vi "icListenHF.vi"() -> ()   [LabVIEW 2020]
uses:
  SubVIs/PAM Reset Array.vi
  SubVIs/icListen 3 Reset.vi
  SubVIs/icListen 2 Reset.vi
  SubVIs/icListen 4 Reset.vi
  SubVIs/icListen 1 Reset.vi
  SubVIs/icListen 2 Connected.vi
  SubVIs/icListen 4 Connected.vi
  SubVIs/icListen 3 Connected.vi
  SubVIs/icListen 1 Connected.vi
  SubVIs/icListen 3 Enabled.vi
  SubVIs/icListen 2 Enabled.vi
  SubVIs/icListen 4 Enabled.vi
  SubVIs/icListen 1 Enabled.vi
  SubVIs/icListen 2 Initialized.vi
  SubVIs/icListen 4 Initialized.vi
  SubVIs/icListen 3 Initialized.vi
  SubVIs/icListen 1 Initialized.vi
  SubVIs/icListen 4 Synchronization.vi
  SubVIs/icListen 3 Synchronization.vi
  SubVIs/icListen 2 Synchronization.vi
  SubVIs/icListen 1 Synchronization.vi
  SubVIs/icListen 4 Serial Number.vi
  SubVIs/icListen 3 Serial Number.vi
  SubVIs/icListen 2 Serial Number.vi
  SubVIs/icListen 1 Serial Number.vi
  SubVIs/PAM Sample Rate.vi
  SubVIs/icListen 1 Position.vi
  SubVIs/icListen 2 Position.vi
  SubVIs/icListen 3 Position.vi
  SubVIs/icListen 4 Position.vi
  SubVIs/PAM Array Buffer Size.vi
  SubVIs/icListen 1 Response.vi
  SubVIs/icListen 2 Response.vi
  SubVIs/icListen 3 Response.vi
  SubVIs/icListen 1 Metadata.vi
  SubVIs/icListen 2 Metadata.vi
  SubVIs/icListen 3 Metadata.vi
  SubVIs/icListen 4 Response.vi
  SubVIs/icListen 4 Metadata.vi
  PAM Library.lvlib
  SubVIs/PAM Volts per Bit.vi
panel:
  out "SN 4":string
  out "SN 3":string
  out "SN 2":string
  out "SN 1":string
  in  "Pos 4":string="Aft Right"
  in  "Pos 3":string="Aft Left"
  in  "Pos 2":string="Fore Right"
  in  "Pos 1":string="Fore Left"
  in  "Sample Rate":T1(ring)=enum."512000"
  in  "Stop":bool
  out "Y min":dbl format="%0.2f"
  out "Y max":dbl format="%0.2f"
  out "size(s) 2":i32
  out "size(s)":i32
  out "Waveform Chart":waveform(dbl)(graph)
  out "Error Out 2":errorcluster
  in  "Error In":errorcluster
  out "TCP IDs 4":T2
  in  "Reset\nArray":bool
  in  "Enable icListen 4":bool
  in  "Enable icListen 3":bool
  in  "Enable icListen 2":bool
  in  "Enable icListen 1":bool=TRUE
  out "Temp":dbl format="%.1g"
  out "Time":string
  out "Status":string="Disabled"
  out "Date":string
  out "Humid":dbl format="%.1g"
  in  "Reset \nicListen 4":bool
  out "Temp":dbl format="%.1g"
  out "Time":string
  out "Temp":dbl format="%.1g"
  out "Time":string
  out "Status":string="Disabled"
  out "Status":string="Disabled"
  out "Temp":dbl format="%.1g"
  out "Time":string
  out "Date":string
  out "Date":string
  out "Date":string
  out "Humid":dbl format="%.1g"
  out "Humid":dbl format="%.1g"
  out "Humid":dbl format="%.1g"
  out "Status":string="Disabled"
  in  "Reset \nicListen 3":bool
  in  "Reset \nicListen 2":bool
  out "TCP IDs 3":T2
  out "TCP IDs 2":T2
  out "Display":waveform(dbl)[](graph)
  out "TCP IDs 1":T2
  out "Error Out":errorcluster
  out "Reset Varibles":errorcluster
  in  "Reset \nicListen 1":bool
  # "Hydrophone Array"
  # "Status & Controls"
  # "Sample Rate [Hz]"
  # "Position"
  # "Status"
  # "Time"
  # "Date"
  # "Temp."
  # "Humid."
  # "SN"
  # "icListen 1"
  # "icListen 2"
  # "icListen 3"
  # "icListen 4"
  # "icListen 1 (SN 1243, Fore Left)"
  # "icListen 2 (SN 1243, Fore Right)"
  # "icListen 3 (SN 1242, Aft Left)"
  # "icListen 4 (SN 1244, Aft Right)"
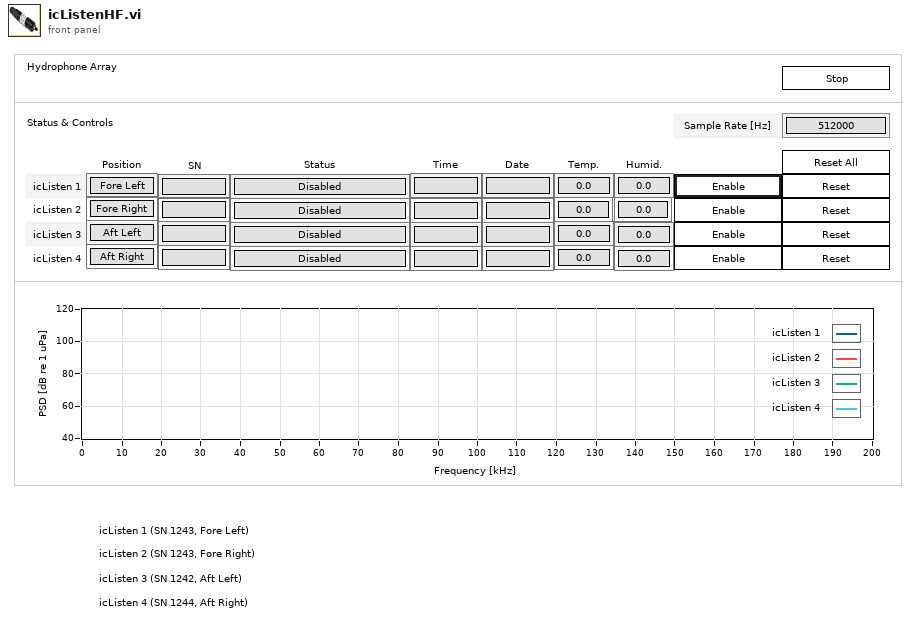
[diagram p1: front panel]
types:
  T1 = enum32{"16000", "32000", "64000", "128000", "256000", "512000"}
  T2 = cluster{"CC Id":refnum<k5>, "Waveform ID":refnum<k5>, "Spectrum ID":refnum<k5>, "Other Data ID":refnum<k5>}
  T3 = cluster{"default (0 U32) 2":i16, "default (0 U32)":i32, "unsigned 64bit integer":u64}
  T4 = cluster{"System Time Status":u8, "Sync Status":u8, "PPS Count":u32, "Sync Offset":u32}
  T5 = cluster{"default (0 U32) 2":i16, "default (0 U32)":i32, "unsigned 64bit integer":u64}[]
  T6 = cluster{"Date":string, "Time":string, "Temperature":dbl, "Humidity":dbl, "Battery Charge":i32}
  T7 = cluster{"State":enum16{"Align with Stream", "Read Header Byte", "Read Data Header", "Read Event Header", "Read Notification", "Read Data"}, "Sample Count":i32, "Timestamp":u64, "Payload":u16, "Repeated Error":i32, "Header Byte":string}
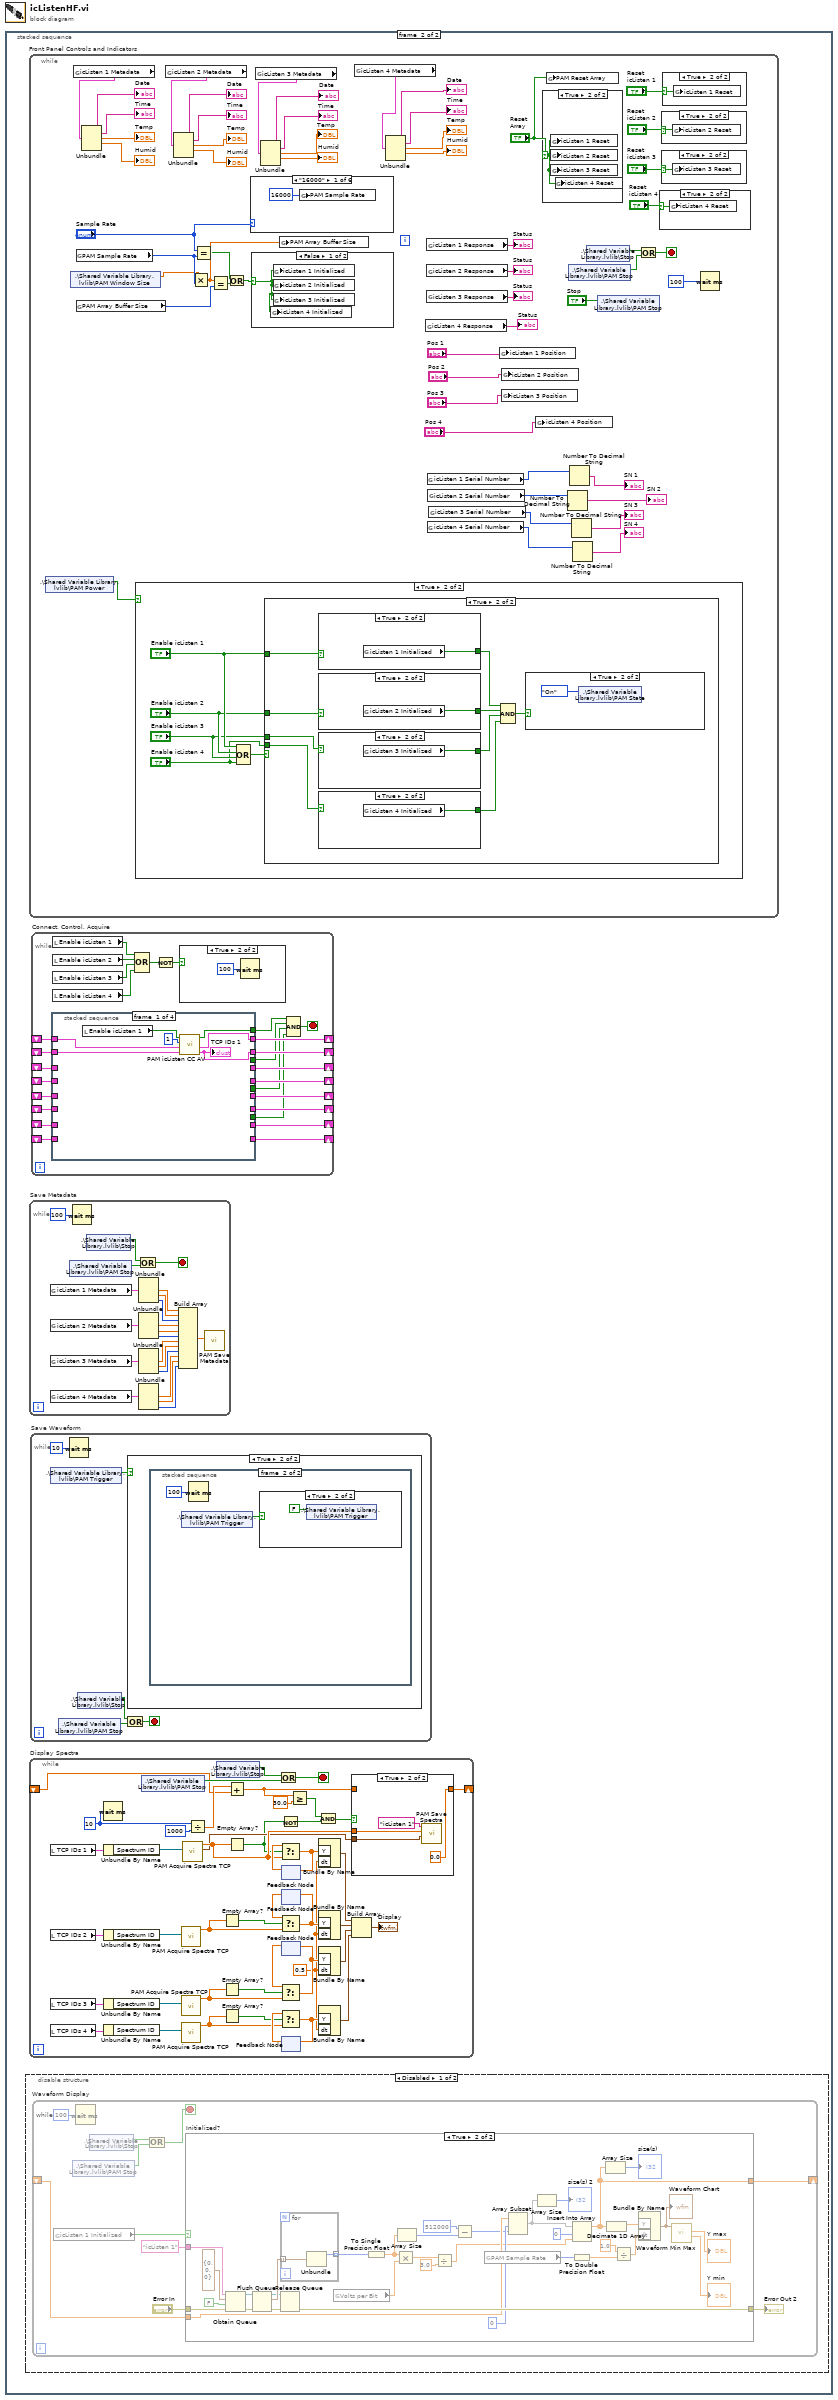
[diagram p0: block diagram]
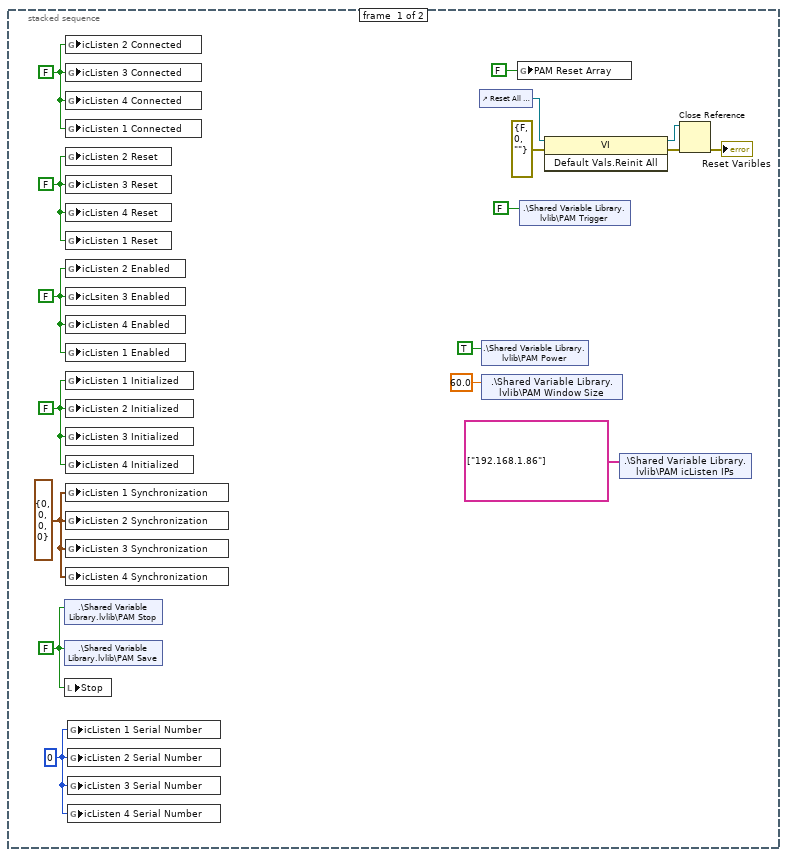
[diagram p2: hidden frame]
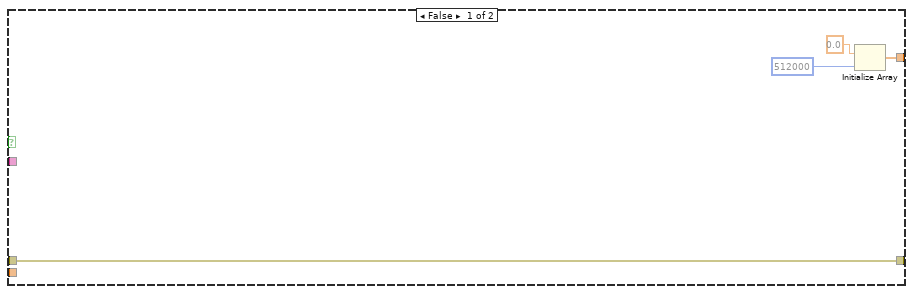
[diagram p4: hidden frame]
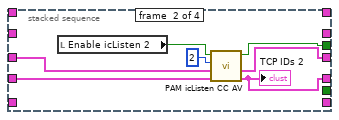
[diagram p7: hidden frame]
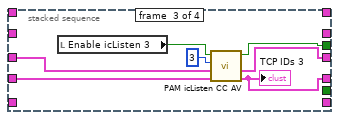
[diagram p8: hidden frame]
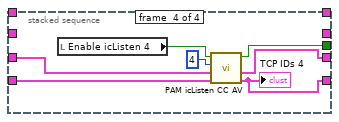
[diagram p9: hidden frame]
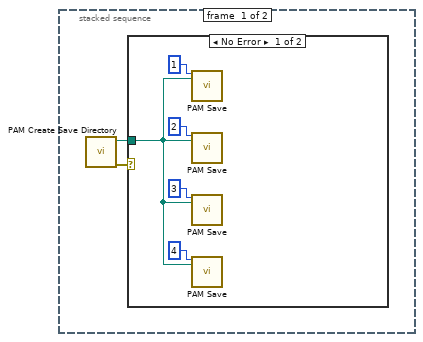
[diagram p11: hidden frame]
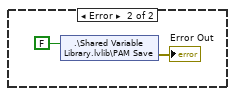
[diagram p12: hidden frame]
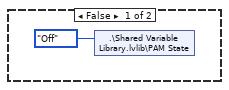
[diagram p14: hidden frame]
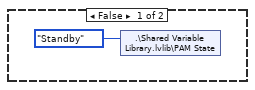
[diagram p15: hidden frame]
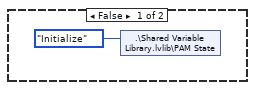
[diagram p16: hidden frame]
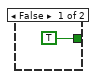
[diagram p17: hidden frame]
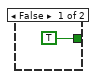
[diagram p18: hidden frame]
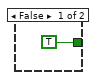
[diagram p19: hidden frame]
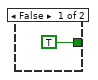
[diagram p20: hidden frame]
diagram:
  n1 = stacked-sequence {
    frame #0 {
      w4 = u16 0 ("icListen 1 Serial Number")
      w6 = FALSE ("PAM Save")
      w8 = T4 {"System Time Status"=0, "Sync Status"=0, "PPS Count"=0, "Sync Offset"=0} ("icListen 1 Synchronization")
      w13 = FALSE ("PAM Stop VI")
      w12 = FALSE ("PAM Stop VI")
      w11 = FALSE ("PAM Stop VI")
      w10 = FALSE ("PAM Stop VI")
      n2 = shared-variable ".\\Shared Variable Library.lvlib\\PAM Stop"(w6) -> ()  [unwired: 1 in, 1 out]
      n3 = shared-variable ".\\Shared Variable Library.lvlib\\PAM Save"(w6) -> ()  [unwired: 1 in, 1 out]
      n4 = local write "Stop"(w6) -> ()
      n5 = global write "icListen 2 Connected.vi" "icListen 2 Connected"(w11) -> ()
      n6 = global write "icListen 3 Connected.vi" "icListen 3 Connected"(w11) -> ()
      n7 = global write "icListen 4 Connected.vi" "icListen 4 Connected"(w11) -> ()
      n8 = global write "icListen 1 Connected.vi" "icListen 1 Connected"(w11) -> ()
      n9 = global write "icListen 2 Reset.vi" "icListen 2 Reset"(w10) -> ()
      n10 = global write "icListen 3 Reset.vi" "icListen 3 Reset"(w10) -> ()
      n11 = global write "icListen 4 Reset.vi" "icListen 4 Reset"(w10) -> ()
      n12 = global write "icListen 1 Reset.vi" "icListen 1 Reset"(w10) -> ()
      n13 = global write "icListen 2 Enabled.vi" "icListen 2 Enabled"(w12) -> ()
      n14 = global write "icListen 3 Enabled.vi" "icLsiten 3 Enabled"(w12) -> ()
      n15 = global write "icListen 4 Enabled.vi" "icListen 4 Enabled"(w12) -> ()
      n16 = global write "icListen 1 Enabled.vi" "icListen 1 Enabled"(w12) -> ()
      n17 = global write "icListen 1 Initialized.vi" "icListen 1 Initialized"(w13) -> ()
      n18 = global write "icListen 2 Initialized.vi" "icListen 2 Initialized"(w13) -> ()
      n19 = global write "icListen 3 Initialized.vi" "icListen 3 Initialized"(w13) -> ()
      n20 = global write "icListen 4 Initialized.vi" "icListen 4 Initialized"(w13) -> ()
      n21 = global write "icListen 1 Synchronization.vi" "icListen 1 Synchronization"(w8) -> ()
      n22 = global write "icListen 2 Synchronization.vi" "icListen 2 Synchronization"(w8) -> ()
      n23 = global write "icListen 3 Synchronization.vi" "icListen 3 Synchronization"(w8) -> ()
      n24 = global write "icListen 4 Synchronization.vi" "icListen 4 Synchronization"(w8) -> ()
      n25 = global write "icListen 1 Serial Number.vi" "icListen 1 Serial Number"(w4) -> ()
      n26 = global write "icListen 2 Serial Number.vi" "icListen 2 Serial Number"(w4) -> ()
      n27 = global write "icListen 3 Serial Number.vi" "icListen 3 Serial Number"(w4) -> ()
      n28 = global write "icListen 4 Serial Number.vi" "icListen 4 Serial Number"(w4) -> ()
      n29 = control-ref of="Reset All VI Variables"() -> (w14:refnum<vi>)
      n30 = shared-variable ".\\Shared Variable Library.lvlib\\PAM Power"(TRUE ("PAM Power")) -> ()  [unwired: 1 in, 1 out]
      n31 = shared-variable ".\\Shared Variable Library.lvlib\\PAM Window Size"(60.0 ("PAM Window Size")) -> ()  [unwired: 1 in, 1 out]
      n32 = global write "PAM Reset Array.vi" "PAM Reset Array"(FALSE ("PAM Stop VI")) -> ()
      n33 = shared-variable ".\\Shared Variable Library.lvlib\\PAM Trigger"(FALSE ("PAM Trigger")) -> ()  [unwired: 1 in, 1 out]
      n34 = invoke class="VI" method="Default Vals.Reinit All"(reference=w14, error in=errorcluster {"status"=FALSE, "code"=0, "source"=""} ("error in (no error)")) -> (reference out=w9:refnum<vi>, error out=w17:errorcluster)  [unwired: 1 in, 1 out]
      n35 = shared-variable ".\\Shared Variable Library.lvlib\\PAM icListen IPs"(string[] ["192.168.1.86"] ("PAM icListen IPs")) -> ()  [unwired: 1 in, 1 out]
      n36 = Close Reference(reference=w9, error in (no error)=w17) -> (error out=→"Reset Varibles":errorcluster)
    }
    frame #1 {
      n37 = disable-structure shown="Disabled" {
        frame Disabled {
          n38 = while "Waveform Display" {
            shift-right: [w73] -> _
            shift-left: _ -> [w72]
            stop <- w74 stop-if-true
            n39 = global read "icListen 1 Initialized.vi" "icListen 1 Initialized"() -> (w69:bool)
            n40 = shared-variable ".\\Shared Variable Library.lvlib\\PAM Stop"() -> (w75:bool)  [unwired: 1 in, 1 out]
            n41 = Wait (ms)(milliseconds to wait=u32 100) -> ()  [unwired: 1 out]
            n42 = shared-variable ".\\Shared Variable Library.lvlib\\Stop"() -> (w76:bool)  [unwired: 1 in, 1 out]
            n43 = Compound Arithmetic op=OR(w76, w75) -> (w74:bool)
            n44 = case "Initialized?" shown="True" w69 {
              tunnel: "Error In" -> [w80 w109]
              tunnel: [w80 w98] -> w71
              tunnel: "icListen 1" ("name (unnamed)") -> [_ w114]
              tunnel: [w77 w85] -> w73
              tunnel: w72 -> [_ w97]
              frame False {
                n45 = Initialize Array(0.0, 512000 ("index")) -> (w77:dbl[])
              }
              frame True {
                n46 = Obtain Queue(name (unnamed)=w114, element data type=T3 {"default (0 U32) 2"=0, "default (0 U32)"=0, "unsigned 64bit integer"=0} ("output cluster"), create if not found? (T)=FALSE, error in (no error)=w109) -> (queue out=w107:refnum<queue>, error out=w106:errorcluster)  [unwired: 1 in, 1 out]
                n47 = Flush Queue(queue=w107, error in (no error)=w106) -> (queue out=w100:refnum<queue>, remaining elements=w102:T5, error out=w99:errorcluster)
                n48 = for {
                  tunnel: w102 -> [w116] mode=indexing
                  tunnel: [w115] -> w103 mode=indexing
                  n49 = Unbundle(w116) -> ("default (0 U32) 2"=w115:i16)  [unwired: 2 out]
                }
                n50 = Release Queue(queue=w100, error in (no error)=w99) -> (error out=w98:errorcluster)  [unwired: 1 in, 2 out]
                n51 = global read "PAM Volts per Bit.vi" "Volts per Bit"() -> (w104:dbl)
                n52 = To Single Precision Float(number=w103) -> (single precision float=w95:sgl[])
                n53 = Multiply(x=w95, y=w104) -> (x*y=w96:dbl[])
                n54 = Array Size(array=w95) -> (size(s)=w92:i32)
                n55 = Divide(x=w96, y=3.0) -> (x/y=w87:dbl[])
                n56 = Subtract(x=512000 ("index"), y=w92) -> (x-y=w91:i32)
                n57 = global read "PAM Sample Rate.vi" "PAM Sample Rate"() -> (w108:i32)
                n58 = Array Subset(array=w97, index=0, length=w91) -> (w89:dbl[])
                n59 = Array Size(array=w89) -> (size(s)=→"size(s) 2":i32)
                n60 = Insert Into Array(array=w89, index=0, new element=w87) -> (w85:dbl[])
                n61 = To Double Precision Float(number=w108) -> (double precision float=w112:dbl)
                n62 = Array Size(array=w85) -> (size(s)=→"size(s)":i32)
                n63 = Decimate 1D Array(w85) -> (w84:dbl[])  [unwired: 1 out]
                n64 = Divide(x=1.0, y=w112) -> (x/y=w113:dbl)
                n65 = Bundle By Name("Y"=w84, "dt"=w113) -> (w83:waveform(dbl))  [unwired: 1 in]
                "Waveform Chart" <- w83
                n66 = call <vilib>:"Waveform Min Max.vi"("waveform in"=w83) -> ("Y min"=→"Y min":dbl, "Y max"=→"Y max":dbl)  [unwired: 5 in, 4 out]
              }
            }
            "Error Out 2" <- w71
          }
        }
        frame Enabled {
        }
      }
      n67 = while "Front Panel Controls and Indicators" {
        stop <- w234 stop-if-true
        n68 = shared-variable ".\\Shared Variable Library.lvlib\\PAM Power"() -> (w224:bool)  [unwired: 1 in, 1 out]
        n69 = shared-variable ".\\Shared Variable Library.lvlib\\PAM Window Size"() -> (w223:dbl)  [unwired: 1 in, 1 out]
        n70 = global read "icListen 1 Metadata.vi" "icListen 1 Metadata"() -> (w242:T6)
        n71 = global read "PAM Sample Rate.vi" "PAM Sample Rate"() -> (w251:i32)
        n72 = global read "PAM Array Buffer Size.vi" "PAM Array Buffer Size"() -> (w263:i32)
        n73 = Unbundle(w242) -> ("Date"=→"Date":string, "Time"=→"Time":string, "Temperature"=→"Temp":dbl, "Humidity"=→"Humid":dbl)  [unwired: 1 out]
        n74 = case shown="True" w224 {
          frame False {
            n75 = shared-variable ".\\Shared Variable Library.lvlib\\PAM State"(enum16{"Off", "Initialize", "On", "Standby"}."Off" ("PAM State")) -> ()  [unwired: 1 in, 1 out]
          }
          frame True {
            n76 = Compound Arithmetic op=OR("Enable icListen 1", "Enable icListen 2", "Enable icListen 3", "Enable icListen 4") -> (w267:bool)
            n77 = case shown="True" w267 {
              tunnel: "Enable icListen 1" -> [_ w281]
              tunnel: "Enable icListen 2" -> [_ w280]
              tunnel: "Enable icListen 3" -> [_ w279]
              tunnel: "Enable icListen 4" -> [_ w278]
              frame False {
                n78 = shared-variable ".\\Shared Variable Library.lvlib\\PAM State"(enum16{"Off", "Initialize", "On", "Standby"}."Standby" ("PAM State")) -> ()  [unwired: 1 in, 1 out]
              }
              frame True {
                n79 = case shown="True" w281 {
                  tunnel: [TRUE ("icListen 1 Initialized") w291] -> w276
                  frame False {
                  }
                  frame True {
                    n80 = global read "icListen 1 Initialized.vi" "icListen 1 Initialized"() -> (w291:bool)
                  }
                }
                n81 = case shown="True" w280 {
                  tunnel: [TRUE ("icListen 1 Initialized") w289] -> w275
                  frame False {
                  }
                  frame True {
                    n82 = global read "icListen 2 Initialized.vi" "icListen 2 Initialized"() -> (w289:bool)
                  }
                }
                n83 = case shown="True" w279 {
                  tunnel: [TRUE ("icListen 1 Initialized") w287] -> w274
                  frame False {
                  }
                  frame True {
                    n84 = global read "icListen 3 Initialized.vi" "icListen 3 Initialized"() -> (w287:bool)
                  }
                }
                n85 = case shown="True" w278 {
                  tunnel: [TRUE ("icListen 1 Initialized") w285] -> w273
                  frame False {
                  }
                  frame True {
                    n86 = global read "icListen 4 Initialized.vi" "icListen 4 Initialized"() -> (w285:bool)
                  }
                }
                n87 = Compound Arithmetic op=AND(w276, w275, w274, w273) -> (w277:bool)
                n88 = case shown="True" w277 {
                  frame False {
                    n89 = shared-variable ".\\Shared Variable Library.lvlib\\PAM State"(enum16{"Off", "Initialize", "On", "Standby"}."Initialize" ("PAM State")) -> ()  [unwired: 1 in, 1 out]
                  }
                  frame True {
                    n90 = shared-variable ".\\Shared Variable Library.lvlib\\PAM State"(enum16{"Off", "Initialize", "On", "Standby"}."On" ("PAM State")) -> ()  [unwired: 1 in, 1 out]
                  }
                }
              }
            }
          }
        }
        n91 = global read "icListen 2 Metadata.vi" "icListen 2 Metadata"() -> (w243:T6)
        n92 = Unbundle(w243) -> ("Date"=→"Date":string, "Time"=→"Time":string, "Temperature"=→"Temp":dbl, "Humidity"=→"Humid":dbl)  [unwired: 1 out]
        n93 = Multiply(x=w223, y=w251) -> (x*y=w264:dbl)
        n94 = Equal?(x="Sample Rate", y=w251) -> (x = y?=w262:bool)
        n95 = Equal?(x=w264, y=w263) -> (x = y?=w260:bool)
        n96 = Or(x=w262, y=w260) -> (x .or. y?=w261:bool)
        n97 = case shown="\"16000\"" "Sample Rate" {
          frame "16000" {
            n98 = global write "PAM Sample Rate.vi" "PAM Sample Rate"(16000 ("PAM Sample Rate")) -> ()
          }
          frame "32000" {
            n99 = global write "PAM Sample Rate.vi" "PAM Sample Rate"(32000 ("PAM Sample Rate")) -> ()
          }
          frame "64000", Default {
            n100 = global write "PAM Sample Rate.vi" "PAM Sample Rate"(64000 ("PAM Sample Rate")) -> ()
          }
          frame "128000" {
            n101 = global write "PAM Sample Rate.vi" "PAM Sample Rate"(128000 ("PAM Sample Rate")) -> ()
          }
          frame "256000" {
            n102 = global write "PAM Sample Rate.vi" "PAM Sample Rate"(256000 ("PAM Sample Rate")) -> ()
          }
          frame "512000" {
            n103 = global write "PAM Sample Rate.vi" "PAM Sample Rate"(512000 ("PAM Sample Rate")) -> ()
          }
        }
        n104 = case shown="False" w261 {
          selector: w261 -> [w297 _]
          frame False {
            n105 = global write "icListen 4 Initialized.vi" "icListen 4 Initialized"(w297) -> ()
            n106 = global write "icListen 1 Initialized.vi" "icListen 1 Initialized"(w297) -> ()
            n107 = global write "icListen 2 Initialized.vi" "icListen 2 Initialized"(w297) -> ()
            n108 = global write "icListen 3 Initialized.vi" "icListen 3 Initialized"(w297) -> ()
          }
          frame True {
          }
        }
        n109 = global read "icListen 3 Metadata.vi" "icListen 3 Metadata"() -> (w244:T6)
        n110 = Unbundle(w244) -> ("Date"=→"Date":string, "Time"=→"Time":string, "Temperature"=→"Temp":dbl, "Humidity"=→"Humid":dbl)  [unwired: 1 out]
        n111 = global write "PAM Array Buffer Size.vi" "PAM Array Buffer Size"(w264) -> ()
        n112 = global read "icListen 4 Metadata.vi" "icListen 4 Metadata"() -> (w230:T6)
        n113 = Unbundle(w230) -> ("Date"=→"Date":string, "Time"=→"Time":string, "Temperature"=→"Temp":dbl, "Humidity"=→"Humid":dbl)  [unwired: 1 out]
        n114 = global read "icListen 4 Response.vi" "icListen 4 Response"() -> (→"Status":string)
        n115 = global read "icListen 1 Response.vi" "icListen 1 Response"() -> (→"Status":string)
        n116 = global read "icListen 2 Response.vi" "icListen 2 Response"() -> (→"Status":string)
        n117 = global read "icListen 3 Response.vi" "icListen 3 Response"() -> (→"Status":string)
        n118 = global read "icListen 1 Serial Number.vi" "icListen 1 Serial Number"() -> (w222:u16)
        n119 = global read "icListen 4 Serial Number.vi" "icListen 4 Serial Number"() -> (w219:u16)
        n120 = global read "icListen 2 Serial Number.vi" "icListen 2 Serial Number"() -> (w221:u16)
        n121 = global read "icListen 3 Serial Number.vi" "icListen 3 Serial Number"() -> (w220:u16)
        n122 = global write "icListen 1 Position.vi" "icListen 1 Position"("Pos 1") -> ()
        n123 = global write "icListen 3 Position.vi" "icListen 3 Position"("Pos 3") -> ()
        n124 = global write "icListen 2 Position.vi" "icListen 2 Position"("Pos 2") -> ()
        n125 = global write "icListen 4 Position.vi" "icListen 4 Position"("Pos 4") -> ()
        n126 = case shown="True" "Reset\nArray" {
          selector: "Reset\nArray" -> [_ w296]
          frame False {
            # "Do Nothing"
          }
          frame True {
            # "Send Reset Command"
            n127 = global write "icListen 1 Reset.vi" "icListen 1 Reset"(w296) -> ()
            n128 = global write "icListen 2 Reset.vi" "icListen 2 Reset"(w296) -> ()
            n129 = global write "icListen 3 Reset.vi" "icListen 3 Reset"(w296) -> ()
            n130 = global write "icListen 4 Reset.vi" "icListen 4 Reset"(w296) -> ()
          }
        }
        n131 = global write "PAM Reset Array.vi" "PAM Reset Array"("Reset\nArray") -> ()
        n132 = Number To Decimal String(number=w221) -> (decimal integer string=→"SN 2":string)  [unwired: 1 in]
        n133 = shared-variable ".\\Shared Variable Library.lvlib\\PAM Stop"() -> (w233:bool)  [unwired: 1 in, 1 out]
        n134 = Number To Decimal String(number=w222) -> (decimal integer string=→"SN 1":string)  [unwired: 1 in]
        n135 = Number To Decimal String(number=w220) -> (decimal integer string=→"SN 3":string)  [unwired: 1 in]
        n136 = Number To Decimal String(number=w219) -> (decimal integer string=→"SN 4":string)  [unwired: 1 in]
        n137 = shared-variable ".\\Shared Variable Library.lvlib\\Stop"() -> (w256:bool)  [unwired: 1 in, 1 out]
        n138 = shared-variable ".\\Shared Variable Library.lvlib\\PAM Stop"("Stop") -> ()  [unwired: 1 in, 1 out]
        n139 = Compound Arithmetic op=OR(w256, w233) -> (w234:bool)
        n140 = case shown="True" "Reset \nicListen 4" {
          selector: "Reset \nicListen 4" -> [_ w292]
          frame False {
          }
          frame True {
            n141 = global write "icListen 4 Reset.vi" "icListen 4 Reset"(w292) -> ()
          }
        }
        n142 = case shown="True" "Reset \nicListen 2" {
          selector: "Reset \nicListen 2" -> [_ w294]
          frame False {
          }
          frame True {
            n143 = global write "icListen 2 Reset.vi" "icListen 2 Reset"(w294) -> ()
          }
        }
        n144 = case shown="True" "Reset \nicListen 3" {
          selector: "Reset \nicListen 3" -> [_ w293]
          frame False {
          }
          frame True {
            n145 = global write "icListen 3 Reset.vi" "icListen 3 Reset"(w293) -> ()
          }
        }
        n146 = case shown="True" "Reset \nicListen 1" {
          selector: "Reset \nicListen 1" -> [_ w295]
          frame False {
          }
          frame True {
            n147 = global write "icListen 1 Reset.vi" "icListen 1 Reset"(w295) -> ()
          }
        }
        n148 = Wait (ms)(milliseconds to wait=u32 100) -> ()  [unwired: 1 out]
      }
      n149 = while "Save Metadata" {
        stop <- w177 stop-if-true
        n150 = global read "icListen 1 Metadata.vi" "icListen 1 Metadata"() -> (w181:T6)
        n151 = global read "icListen 2 Metadata.vi" "icListen 2 Metadata"() -> (w182:T6)
        n152 = global read "icListen 3 Metadata.vi" "icListen 3 Metadata"() -> (w183:T6)
        n153 = global read "icListen 4 Metadata.vi" "icListen 4 Metadata"() -> (w176:T6)
        n154 = shared-variable ".\\Shared Variable Library.lvlib\\PAM Stop"() -> (w178:bool)  [unwired: 1 in, 1 out]
        n155 = Wait (ms)(milliseconds to wait=u32 100) -> ()  [unwired: 1 out]
        n156 = shared-variable ".\\Shared Variable Library.lvlib\\Stop"() -> (w179:bool)  [unwired: 1 in, 1 out]
        n157 = Unbundle(w181) -> ("Temperature"=w184:dbl, "Humidity"=w185:dbl, "Battery Charge"=w186:i32)  [unwired: 2 out]
        n158 = Unbundle(w182) -> ("Temperature"=w187:dbl, "Humidity"=w188:dbl, "Battery Charge"=w189:i32)  [unwired: 2 out]
        n159 = Unbundle(w183) -> ("Temperature"=w190:dbl, "Humidity"=w191:dbl, "Battery Charge"=w192:i32)  [unwired: 2 out]
        n160 = Unbundle(w176) -> ("Temperature"=w175:dbl, "Humidity"=w174:dbl, "Battery Charge"=w173:i32)  [unwired: 2 out]
        n161 = Compound Arithmetic op=OR(w179, w178) -> (w177:bool)
        n162 = Build Array(w184, w185, w186, w187, w188, w189, w190, w191, w192, w175, w174, w173) -> (w180:dbl[])
        n163 = call "PAM Save Metadata.vi"("Values"=w180) -> ()  [unwired: 9 in]
      }
      n164 = while "Display Spectra" {
        shift-right: [w18] -> _
        shift-left: _ -> [w19]
        stop <- w59 stop-if-true
        w31 = 0.5 ("dt")
        w28 = u32 10 ("milliseconds to wait")
        n165 = local read "TCP IDs 1"() -> (w58:T2)
        n166 = local read "TCP IDs 2"() -> (w49:T2)
        n167 = local read "TCP IDs 3"() -> (w48:T2)
        n168 = local read "TCP IDs 4"() -> (w35:T2)
        n169 = Wait (ms)(milliseconds to wait=w28) -> ()  [unwired: 1 out]
        n170 = Unbundle By Name(w58) -> ("Spectrum ID"=w39:refnum<k5>)
        n171 = Unbundle By Name(w49) -> ("Spectrum ID"=w41:refnum<k5>)
        n172 = Unbundle By Name(w48) -> ("Spectrum ID"=w40:refnum<k5>)
        n173 = Unbundle By Name(w35) -> ("Spectrum ID"=w38:refnum<k5>)
        n174 = shared-variable ".\\Shared Variable Library.lvlib\\PAM Stop"() -> (w60:bool)  [unwired: 1 in, 1 out]
        n175 = call "PAM Acquire Spectra TCP.vi"("Spectrum ID"=w41) -> ("PSD Out"=w47:dbl[])  [unwired: 9 in, 1 out]
        n176 = call "PAM Acquire Spectra TCP.vi"("Spectrum ID"=w40) -> ("PSD Out"=w50:dbl[])  [unwired: 9 in, 1 out]
        n177 = call "PAM Acquire Spectra TCP.vi"("Spectrum ID"=w38) -> ("PSD Out"=w34:dbl[])  [unwired: 9 in, 1 out]
        n178 = call "PAM Acquire Spectra TCP.vi"("Spectrum ID"=w39) -> ("Timestamp Out"=w29:timestamp, "PSD Out"=w30:dbl[])  [unwired: 9 in]
        n179 = Divide(x=w28, y=u32 1000) -> (x/y=w26:dbl)
        n180 = shared-variable ".\\Shared Variable Library.lvlib\\Stop"() -> (w61:bool)  [unwired: 1 in, 1 out]
        n181 = Empty Array?(array=w47) -> (empty?=w52:bool)
        n182 = Empty Array?(array=w50) -> (empty?=w51:bool)
        n183 = Empty Array?(array=w34) -> (empty?=w33:bool)
        n184 = Add(x=w26, y=w19) -> (x+y=w20:dbl)
        n185 = Empty Array?(array=w30) -> (empty?=w21:bool)
        n186 = Not(x=w21) -> (.not. x?=w22:bool)
        n187 = Compound Arithmetic op=OR(w61, w60) -> (w59:bool)
        n188 = feedback #1() -> (w53:dbl[])  [unwired: 1 in]
        n189 = Select(t=w53, s=w21, f=w30) -> (s? t:f=w43:dbl[])
        n190 = feedback-in #1(w43) -> ()
        n191 = feedback #2() -> (w46:dbl[])  [unwired: 1 in]
        n192 = Select(t=w46, s=w52, f=w47) -> (s? t:f=w42:dbl[])
        n193 = feedback-in #2(w42) -> ()
        n194 = feedback #3() -> (w45:dbl[])  [unwired: 1 in]
        n195 = Select(t=w45, s=w51, f=w50) -> (s? t:f=w44:dbl[])
        n196 = feedback-in #3(w44) -> ()
        n197 = feedback #4() -> (w36:dbl[])  [unwired: 1 in]
        n198 = Select(t=w36, s=w33, f=w34) -> (s? t:f=w37:dbl[])
        n199 = feedback-in #4(w37) -> ()
        n200 = Greater Or Equal?(x=w20, y=30.0) -> (x >= y?=w24:bool)
        n201 = And(x=w24, y=w22) -> (x .and. y?=w23:bool)
        n202 = Bundle By Name("Y"=w43, "dt"=w31) -> (w57:waveform(dbl))  [unwired: 1 in]
        n203 = Bundle By Name("Y"=w42, "dt"=w31) -> (w56:waveform(dbl))  [unwired: 1 in]
        n204 = Bundle By Name("Y"=w44, "dt"=w31) -> (w55:waveform(dbl))  [unwired: 1 in]
        n205 = Bundle By Name("Y"=w37, "dt"=w31) -> (w32:waveform(dbl))  [unwired: 1 in]
        n206 = case shown="True" w23 {
          tunnel: w30 -> [_ w65]
          tunnel: w29 -> [_ w64]
          tunnel: w20 -> [w62 _]
          tunnel: [w62 0.0] -> w18
          frame False {
          }
          frame True {
            n207 = call "PAM Save Spectra.vi"("Time"=w64, "PSD"=w65, "icListen"="icListen 1") -> ()  [unwired: 9 in]
          }
        }
        n208 = Build Array(w57, w56, w55, w32) -> (→"Display":waveform(dbl)[])
      }
      n209 = while "Save Waveform" {
        stop <- w195 stop-if-true
        n210 = shared-variable ".\\Shared Variable Library.lvlib\\PAM Trigger"() -> (w194:bool)  [unwired: 1 in, 1 out]
        n211 = shared-variable ".\\Shared Variable Library.lvlib\\PAM Stop"() -> (w196:bool)  [unwired: 1 in, 1 out]
        n212 = Wait (ms)(milliseconds to wait=u32 10) -> ()  [unwired: 1 out]
        n213 = shared-variable ".\\Shared Variable Library.lvlib\\Stop"() -> (w197:bool)  [unwired: 1 in, 1 out]
        n214 = case shown="True" w194 {
          frame False {
          }
          frame True {
            n215 = stacked-sequence {
              frame #0 {
                n216 = call "PAM Create Save Directory.vi"() -> ("Error Out"=w200:errorcluster, "Path"=w199:path)  [unwired: 10 in]
                n217 = case shown="No Error" w200 {
                  tunnel: w199 -> [w201 _]
                  frame No Error {
                    n218 = call "PAM Save.vi"("icListen #"=1, "Path"=w201) -> ()  [unwired: 18 in]
                    n219 = call "PAM Save.vi"("icListen #"=2, "Path"=w201) -> ()  [unwired: 18 in]
                    n220 = call "PAM Save.vi"("icListen #"=3, "Path"=w201) -> ()  [unwired: 18 in]
                    n221 = call "PAM Save.vi"("icListen #"=4, "Path"=w201) -> ()  [unwired: 18 in]
                  }
                  frame Error {
                    n222 = shared-variable ".\\Shared Variable Library.lvlib\\PAM Save"(FALSE ("PAM Save")) -> (error out=→"Error Out":errorcluster)  [unwired: 1 in]
                  }
                }
              }
              frame #1 {
                n223 = shared-variable ".\\Shared Variable Library.lvlib\\PAM Trigger"() -> (w209:bool)  [unwired: 1 in, 1 out]
                n224 = Wait (ms)(milliseconds to wait=u32 100) -> ()  [unwired: 1 out]
                n225 = case shown="True" w209 {
                  frame False {
                  }
                  frame True {
                    n226 = shared-variable ".\\Shared Variable Library.lvlib\\PAM Trigger"(FALSE ("PAM Trigger")) -> ()  [unwired: 1 in, 1 out]
                  }
                }
              }
            }
          }
        }
        n227 = Compound Arithmetic op=OR(w197, w196) -> (w195:bool)
      }
      n228 = while "Connect, Control, Acquire" {
        shift-right: [w143] -> _
        shift-left: _ -> [w142]
        shift-right: [w140] -> _
        shift-left: _ -> [w141]
        shift-right: [w139] -> _
        shift-left: _ -> [w138]
        shift-right: [w137] -> _
        shift-left: _ -> [w136]
        shift-right: [w135] -> _
        shift-left: _ -> [w134]
        shift-right: [w133] -> _
        shift-left: _ -> [w132]
        shift-right: [w131] -> _
        shift-left: _ -> [w130]
        shift-right: [w129] -> _
        shift-left: _ -> [w128]
        stop <- w123 stop-if-true
        n229 = stacked-sequence {
          tunnel: w142 -> [w151 _ _ _]
          tunnel: w141 -> [w150 _ _ _]
          tunnel: [w147 _ _ _] -> w143
          tunnel: [w149 _ _ _] -> w140
          tunnel: [_ w158 _ _] -> w139
          tunnel: w138 -> [_ w157 _ _]
          tunnel: [_ w155 _ _] -> w137
          tunnel: w136 -> [_ w156 _ _]
          tunnel: [w148 _ _ _] -> w127
          tunnel: [_ _ w162 _] -> w135
          tunnel: w134 -> [_ _ w165 _]
          tunnel: [_ _ w164 _] -> w133
          tunnel: w132 -> [_ _ w163 _]
          tunnel: [_ _ _ w172] -> w131
          tunnel: w130 -> [_ _ _ w171]
          tunnel: [_ _ _ w170] -> w129
          tunnel: w128 -> [_ _ _ w169]
          tunnel: [_ w154 _ _] -> w126
          tunnel: [_ _ w161 _] -> w125
          tunnel: [_ _ _ w168] -> w124
          frame #0 {
            n230 = local read "Enable icListen 1"() -> (w145:bool)
            n231 = call "PAM icListen CC AV.vi"("TCP IDs In"=w151, "Acq In"=w150, "icListen #"=1, "Enabled"=w145) -> ("TCP IDs Out"=w147:T2, "Acq Out"=w149:T7, "Stop"=w148:bool)  [unwired: 1 in]
            "TCP IDs 1" <- w147
          }
          frame #1 {
            n232 = local read "Enable icListen 2"() -> (w152:bool)
            n233 = call "PAM icListen CC AV.vi"("TCP IDs In"=w156, "Acq In"=w157, "icListen #"=2, "Enabled"=w152) -> ("TCP IDs Out"=w155:T2, "Acq Out"=w158:T7, "Stop"=w154:bool)  [unwired: 1 in]
            "TCP IDs 2" <- w155
          }
          frame #2 {
            n234 = local read "Enable icListen 3"() -> (w159:bool)
            n235 = call "PAM icListen CC AV.vi"("TCP IDs In"=w165, "Acq In"=w163, "icListen #"=3, "Enabled"=w159) -> ("TCP IDs Out"=w162:T2, "Acq Out"=w164:T7, "Stop"=w161:bool)  [unwired: 1 in]
            "TCP IDs 3" <- w162
          }
          frame #3 {
            n236 = local read "Enable icListen 4"() -> (w166:bool)
            n237 = call "PAM icListen CC AV.vi"("TCP IDs In"=w169, "Acq In"=w171, "icListen #"=4, "Enabled"=w166) -> ("TCP IDs Out"=w170:T2, "Acq Out"=w172:T7, "Stop"=w168:bool)  [unwired: 1 in]
            "TCP IDs 4" <- w170
          }
        }
        n238 = local read "Enable icListen 1"() -> (w122:bool)
        n239 = local read "Enable icListen 2"() -> (w121:bool)
        n240 = local read "Enable icListen 3"() -> (w120:bool)
        n241 = local read "Enable icListen 4"() -> (w119:bool)
        n242 = Compound Arithmetic op=OR(w122, w121, w120, w119) -> (w118:bool)
        n243 = Not(x=w118) -> (.not. x?=w117:bool)
        n244 = case shown="True" w117 {
          frame False {
          }
          frame True {
            n245 = Wait (ms)(milliseconds to wait=u32 100) -> ()  [unwired: 1 out]
          }
        }
        n246 = Compound Arithmetic op=AND(w127, w126, w125, w124) -> (w123:bool)
      }
    }
  }
